vi "write_log_file.vi"(8 "error in":errorcluster, 10 "Event log":T1[](array[typedef]) {"Timestamp" format="%<%.3X>T"}, 11 "Log file":path) -> (0 "error out":errorcluster)   [LabVIEW 2012]
uses:
  log_event.ctl
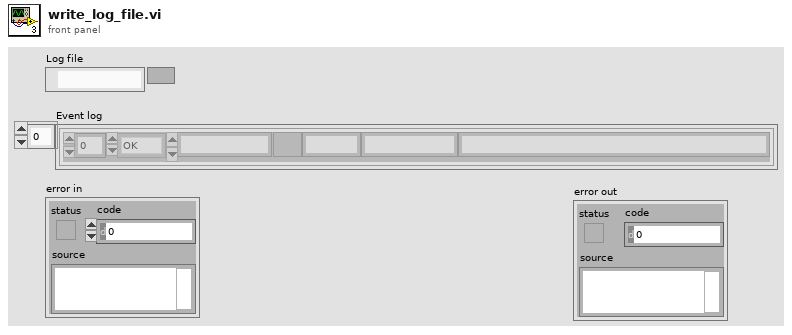
[diagram p1: front panel]
types:
  T1 = typedef "log_event.ctl" = cluster{"Facility ID":i32, "Severity":enum16{"OK", "Debug", "Warn", "Error"}, "Timestamp":timestamp, "Facility":string, "State":string, "Message":string}
  T2 = enum16{"open", "replace", "create", "open or create", "replace or create", "replace or create with confirmation"}
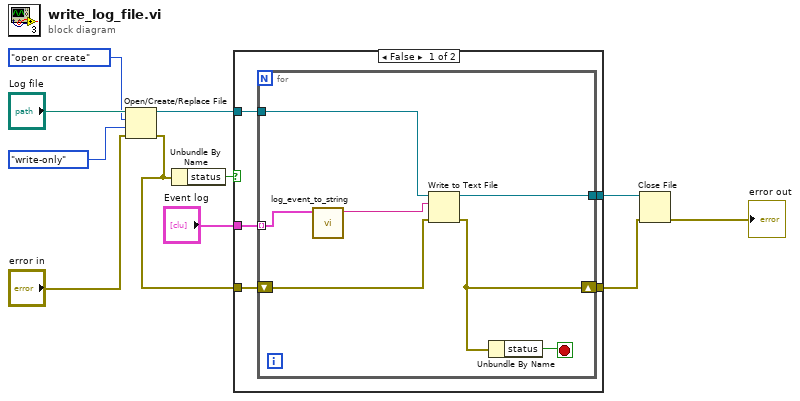
[diagram p0: block diagram]
diagram:
  n1 = Open/Create/Replace File(file path (use dialog)="Log file", error in="error in", operation (0:open)=T2."open or create", access (0:read/write)=enum16{"read/write", "read-only", "write-only"}."write-only") -> (refnum out=w4:refnum<file>, error out=w10:errorcluster)  [unwired: 2 in, 1 out]
  n2 = Unbundle By Name(w10) -> ("status"=w3:bool)
  n3 = case shown="False" w3 {
    tunnel: w4 -> [w15 w25]
    tunnel: "Event log" -> [w16 _]
    tunnel: [w14 w25] -> w7
    tunnel: [w13 w24] -> w8
    tunnel: w10 -> [w12 w24]
    frame False {
      n4 = for {
        tunnel: w16 -> [w22] mode=indexing
        tunnel: w15 -> [w23]
        shift-right: [w19] -> w13
        shift-left: w12 -> [w20]
        tunnel: [w17] -> w14
        stop <- w18 stop-if-true
        n5 = call "log_event_to_string.vi"("Log event"=w22) -> ("String"=w21:string)  [unwired: 10 in]
        n6 = Write to Text File(file (use dialog)=w23, text=w21, error in=w20) -> (refnum out=w17:refnum<file>, error out=w19:errorcluster)  [unwired: 1 in, 1 out]
        n7 = Unbundle By Name(w19) -> ("status"=w18:bool)
      }
    }
    frame True {
    }
  }
  n8 = Close File(refnum=w7, error in=w8) -> (error out=→"error out":errorcluster)  [unwired: 1 out]
